vi "UTILITY AutoScroll DEBUG and BUS.vi"(10 "Input Data":string, 11 "Debug Data":string) -> (2 "Text Scroll Position":i32, 3 "Output Limit":string)   [LabVIEW 2016]
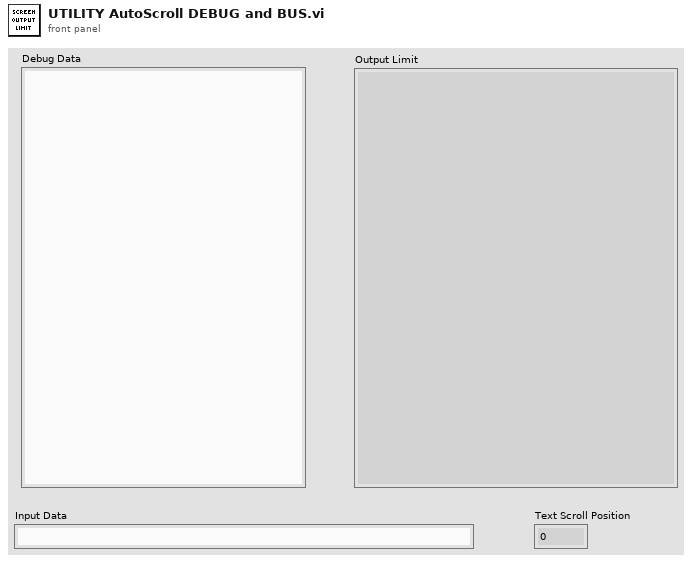
[diagram p1: front panel]
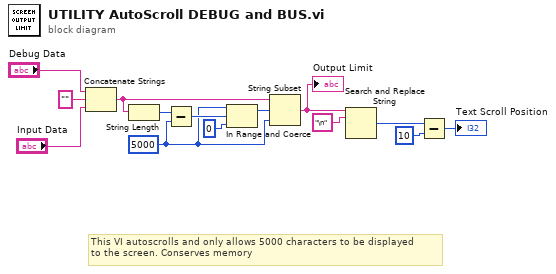
[diagram p0: block diagram]
diagram:
  w4 = 5000 ("length (rest)")
  # "This VI autoscrolls and only allows 5000 characters to be displayed \nto the screen. Conserves memory"
  n1 = Concatenate Strings("Debug Data", "" ("Msg Delimiter"), "Input Data") -> (w2:string)
  n2 = String Length(string=w2) -> (length=w7:i32)
  n3 = Subtract(x=w7, y=w4) -> (x-y=w6:i32)
  n4 = In Range and Coerce(upper limit=w4, x=w6, lower limit=0) -> (coerced(x)=w3:i32)  [unwired: 1 out]
  n5 = String Subset(string=w2, offset (0)=w3, length (rest)=w4) -> (substring=w12:string)
  "Output Limit" <- w12
  n6 = Search and Replace String(input string=w12, search string="\n") -> (number of replacements=w10:i32)  [unwired: 6 in, 3 out]
  n7 = Subtract(x=w10, y=10) -> (x-y=→"Text Scroll Position":i32)
